vi "IMAQ FPGA Camera Link Pixel Packer.vi"   [LabVIEW 2017]
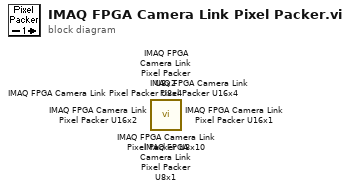
[diagram p0: block diagram]
diagram:
  n1 = call <vilib>:"IMAQ FPGA Camera Link Pixel Packer U8x10.vi"() -> ()  [unwired: 7 in, 5 out]
  n2 = call <vilib>:"IMAQ FPGA Camera Link Pixel Packer U16x4.vi"() -> ()  [unwired: 8 in, 4 out]
  n3 = call <vilib>:"IMAQ FPGA Camera Link Pixel Packer U16x2.vi"() -> ()  [unwired: 8 in, 4 out]
  n4 = call <vilib>:"IMAQ FPGA Camera Link Pixel Packer U16x1.vi"() -> ()  [unwired: 8 in, 4 out]
  n5 = call <vilib>:"IMAQ FPGA Camera Link Pixel Packer U8x4.vi"() -> ()  [unwired: 8 in, 4 out]
  n6 = call <vilib>:"IMAQ FPGA Camera Link Pixel Packer U8x2.vi"() -> ()  [unwired: 8 in, 4 out]
  n7 = call <vilib>:"IMAQ FPGA Camera Link Pixel Packer U8x1.vi"() -> ()  [unwired: 8 in, 4 out]
